vi "RampVoltagewithDDSv12.vi"() -> ()   [LabVIEW 2016]
uses:
  <vilib>/DAQmx/write.llb/DAQmx Write (Digital 1D Wfm NChan NSamp).vi
  <vilib>/DAQmx/write.llb/DAQmx Write (Analog 2D DBL NChan NSamp).vi
  <vilib>/DAQmx/create/channels.llb/DAQmx Create Channel (AO-Voltage-Basic).vi
  <vilib>/DAQmx/create/channels.llb/DAQmx Create Channel (DO-Digital Output).vi
  <vilib>/DAQmx/configure/timing.llb/DAQmx Timing (Sample Clock).vi
  <vilib>/DAQmx/configure/trigger.llb/DAQmx Start Trigger (Digital Edge).vi
  <vilib>/DAQmx/miscellaneous.llb/DAQmx Fill In Error Info.vi
  <vilib>/Waveform/DWDTOps.llb/DWDT Boolean Array to Digital.vi
  <vilib>/Waveform/DWDTOps.llb/DWDT Uncompress Digital.vi
  <vilib>/Waveform/DTblOps.llb/DTbl Digital to Analog.vi
  <resource>/objmgr/daqmx.rc
panel:
  in  "Phase Lock Switch\n(TTL High - Lock Off)":bool
  in  "Phase Lock Switch (Port 0 Line 1)":tag="Dev2/port0/line1"
  out "Digital Output":cluster{i32, dbl, dbl[][]}(graph)={0, 1e-05, [[0.0, 0.0, 0.0, 0.0, 0.0, 0.0, 0.0, 0.0, 0.0, 0.0, 0.0, 0.0, 0.0, 0.0, 0.0, 0.0, 0.0, 0.0, 0.0, 0.0, 0.0, 0.0, 0.0, 0.0, 0.0, 0.0, 0.0, 0.0, 0.0, 0.0, 0.0, 0.0, 0.0, 0.0, 0.0, 0.0, 0.0, 0.0, 0.0, 0.0, 0.0, 0.0, 0.0, 0.0, 0.0, 0.0, 0.0, 0.0, 0.0, 0.0, 0.0, 0.0, 0.0, 0.0, 0.0, 0.0, 0.0, 0.0, 0.0, 0.0, 0.0, 0.0, 0.0, 0.0, 0.0, 0.0, 0.0, 0.0, 0.0, 0.0, 0.0, 0.0, 0.0, 0.0, 0.0, 0.0, 0.0, 0.0, 0.0, 0.0, 0.0, 0.0, 0.0, 0.0, 0.0, 0.0, 0.0, 0.0, 0.0, 0.0, 0.0, 0.0, 0.0, 0.0, 0.0, 0.0, 0.0, 0.0, 0.0, 0.0, 5.0, 5.0, 5.0, 5.0, 5.0, 5.0, 5.0, 5.0, 5.0, 5.0, 5.0, 5.0, 5.0, 5.0, 5.0, 5.0, 5.0, 5.0, 5.0, 5.0, 5.0, 5.0, 5.0, 5.0, 5.0, 5.0, 5.0, 5.0, 5.0, 5.0, 5.0, 5.0, 5.0, 5.0, 5.0, 5.0, 5.0, 5.0, 5.0, 5.0, 5.0, 5.0, 5.0, 5.0, 5.0, 5.0, 5.0, 5.0, 5.0, 5.0, 5.0, 5.0, 5.0, 5.0, 5.0, 5.0, 5.0, 5.0, 5.0, 5.0, 5.0, 5.0, 5.0, 5.0, 5.0, 5.0, 5.0, 5.0, 5.0, 5.0, 5.0, 5.0, 5.0, 5.0, 5.0, 5.0, 5.0, 5.0, 5.0, 5.0, 5.0, 5.0, 5.0, 5.0, 5.0, 5.0, 5.0, 5.0, 5.0, 5.0, 5.0, 5.0, 5.0, 5.0, 5.0, 5.0, 5.0, 5.0, 5.0, 5.0, 5.0, 5.0, 5.0, 5.0, 5.0, 5.0, 5.0, 5.0, 5.0, 5.0, 5.0, 5.0, 5.0, 5.0, 5.0, 5.0, 5.0, 5.0, 5.0, 5.0, 5.0, 5.0, 5.0, 5.0, 5.0, 5.0, 5.0, 5.0, 5.0, 5.0, 5.0, 5.0, 5.0, 5.0, 5.0, 5.0, 5.0, 5.0, 5.0, 5.0, 5.0, 5.0, 5.0, 5.0, 5.0, 5.0, 5.0, 5.0, 5.0, 5.0, 5.0, 5.0, 5.0, 5.0, 5.0, 5.0, 5.0, 5.0, 5.0, 5.0, 5.0, 5.0, 5.0, 5.0, 5.0, 5.0, 5.0, 5.0, 5.0, 5.0, 5.0, 5.0, 5.0, 5.0, 5.0, 5.0, 5.0, 5.0, 5.0, 5.0, 5.0, 5.0, 5.0, 5.0, 5.0, 5.0, 5.0, 5.0, 5.0, 5.0, 5.0, 5.0, 5.0, 5.0, 5.0, 5.0, 5.0, 5.0, 5.0, 5.0, 0.0, 0.0, 0.0, 0.0, 0.0, 0.0, 0.0, 0.0, 0.0, 0.0, 0.0, 0.0, 0.0, 0.0, 0.0, 0.0, 0.0, 0.0, 0.0, 0.0, 0.0, 0.0, 0.0, 0.0, 0.0, 0.0, 0.0, 0.0, 0.0, 0.0, 0.0, 0.0, 0.0, 0.0, 0.0, 0.0, 0.0, 0.0, 0.0, 0.0, 0.0, 0.0, 0.0, 0.0, 0.0, 0.0, 0.0, 0.0, 0.0, 0.0, 0.0, 0.0, 0.0, 0.0, 0.0, 0.0, 0.0, 0.0, 0.0, 0.0, 0.0, 0.0, 0.0, 0.0, 0.0, 0.0, 0.0, 0.0, 0.0, 0.0, 0.0, 0.0, 0.0, 0.0, 0.0, 0.0, 0.0, 0.0, 0.0, 0.0, 0.0, 0.0, 0.0, 0.0, 0.0, 0.0, 0.0, 0.0, 0.0, 0.0, 0.0, 0.0, 0.0, 0.0, 0.0, 0.0, 0.0, 0.0, 0.0, 0.0, 0.0, 0.0, 0.0, 0.0, 0.0, 0.0, 0.0, 0.0, 0.0, 0.0, 0.0, 0.0, 0.0, 0.0, 0.0, 0.0, 0.0, 0.0, 0.0, 0.0, 0.0, 0.0, 0.0, 0.0, 0.0, 0.0, 0.0, 0.0, 0.0, 0.0, 0.0, 0.0, 0.0, 0.0, 0.0, 0.0, 0.0, 0.0, 0.0, 0.0, 0.0, 0.0, 0.0, 0.0, 0.0, 0.0, 0.0, 0.0, 0.0, 0.0, 0.0, 0.0, 0.0, 0.0, 0.0, 0.0, 0.0, 0.0, 0.0, 0.0, 0.0, 0.0, 0.0, 0.0, 0.0, 0.0, 0.0, 0.0, 0.0, 0.0, 0.0, 0.0, 0.0, 0.0, 0.0, 0.0, 0.0, 0.0, 0.0, 0.0, 0.0, 0.0, 0.0, 0.0, 0.0, 0.0, 0.0, 0.0, 0.0, 0.0, 0.0, 0.0, 0.0, 0.0, 0.0, 0.0, 0.0, 0.0, 0.0, 0.0, 5.0, 5.0, 5.0, 5.0, 5.0, 5.0, 5.0, 5.0, 5.0, 5.0, 5.0, 5.0, 5.0, 5.0, 5.0, 5.0, 5.0, 5.0, 5.0, 5.0, 5.0, 5.0, 5.0, 5.0, 5.0, 5.0, 5.0, 5.0, 5.0, 5.0, 5.0, 5.0, 5.0, 5.0, 5.0, 5.0, 5.0, 5.0, 5.0, 5.0, 5.0, 5.0, 5.0, 5.0, 5.0, 5.0, 5.0, 5.0, 5.0, 5.0, 5.0, 5.0, 5.0, 5.0, 5.0, 5.0, 5.0, 5.0, 5.0, 5.0, 5.0, 5.0, 5.0, 5.0, 5.0, 5.0, 5.0, 5.0, 5.0, 5.0, 5.0, 5.0, 5.0, 5.0, 5.0, 5.0, 5.0, 5.0, 5.0, 5.0, 5.0, 5.0, 5.0, 5.0, 5.0, 5.0, 5.0, 5.0, 5.0, 5.0, 5.0, 5.0, 5.0, 5.0, 5.0, 5.0, 5.0, 5.0, 5.0, 5.0, 5.0, 5.0, 5.0, 5.0, 5.0, 5.0, 5.0, 5.0, 5.0, 5.0, 5.0, 5.0, 5.0, 5.0, 5.0, 5.0, 5.0, 5.0, 5.0, 5.0, 5.0, 5.0, 5.0, 5.0, 5.0, 5.0, 5.0, 5.0, 5.0, 5.0, 5.0, 5.0, 5.0, 5.0, 5.0, 5.0, 5.0, 5.0, 5.0, 5.0, 5.0, 5.0, 5.0, 5.0, 5.0, 5.0, 5.0, 5.0, 5.0, 5.0, 5.0, 5.0, 5.0, 5.0, 5.0, 5.0, 5.0, 5.0, 5.0, 5.0, 5.0, 5.0, 5.0, 5.0, 5.0, 5.0, 5.0, 5.0, 5.0, 5.0, 5.0, 5.0, 5.0, 5.0, 5.0, 5.0, 5.0, 5.0, 5.0, 5.0, 5.0, 5.0, 5.0, 5.0, 5.0, 5.0, 5.0, 5.0, 5.0, 5.0, 5.0, 5.0, 5.0, 5.0, 5.0, 5.0, 5.0, 5.0, 5.0, 5.0, 0.0, 0.0, 0.0, 0.0, 0.0, 0.0, 0.0, 0.0, 0.0, 0.0, 0.0, 0.0, 0.0, 0.0, 0.0, 0.0, 0.0, 0.0, 0.0, 0.0, 0.0, 0.0, 0.0, 0.0, 0.0, 0.0, 0.0, 0.0, 0.0, 0.0, 0.0, 0.0, 0.0, 0.0, 0.0, 0.0, 0.0, 0.0, 0.0, 0.0, 0.0, 0.0, 0.0, 0.0, 0.0, 0.0, 0.0, 0.0, 0.0, 0.0, 0.0, 0.0, 0.0, 0.0, 0.0, 0.0, 0.0, 0.0, 0.0, 0.0, 0.0, 0.0, 0.0, 0.0, 0.0, 0.0, 0.0, 0.0, 0.0, 0.0, 0.0, 0.0, 0.0, 0.0, 0.0, 0.0, 0.0, 0.0, 0.0, 0.0, 0.0, 0.0, 0.0, 0.0, 0.0, 0.0, 0.0, 0.0, 0.0, 0.0, 0.0, 0.0, 0.0, 0.0, 0.0, 0.0, 0.0, 0.0, 0.0, 0.0, 5.0], [5.0, 5.0, 5.0, 5.0, 5.0, 5.0, 5.0, 5.0, 5.0, 5.0, 5.0, 5.0, 5.0, 5.0, 5.0, 5.0, 5.0, 5.0, 5.0, 5.0, 5.0, 5.0, 5.0, 5.0, 5.0, 5.0, 5.0, 5.0, 5.0, 5.0, 5.0, 5.0, 5.0, 5.0, 5.0, 5.0, 5.0, 5.0, 5.0, 5.0, 5.0, 5.0, 5.0, 5.0, 5.0, 5.0, 5.0, 5.0, 5.0, 5.0, 5.0, 5.0, 5.0, 5.0, 5.0, 5.0, 5.0, 5.0, 5.0, 5.0, 5.0, 5.0, 5.0, 5.0, 5.0, 5.0, 5.0, 5.0, 5.0, 5.0, 5.0, 5.0, 5.0, 5.0, 5.0, 5.0, 5.0, 5.0, 5.0, 5.0, 5.0, 5.0, 5.0, 5.0, 5.0, 5.0, 5.0, 5.0, 5.0, 5.0, 5.0, 5.0, 5.0, 5.0, 5.0, 5.0, 5.0, 5.0, 5.0, 5.0, 5.0, 5.0, 5.0, 5.0, 5.0, 5.0, 5.0, 5.0, 5.0, 5.0, 5.0, 5.0, 5.0, 5.0, 5.0, 5.0, 5.0, 5.0, 5.0, 5.0, 5.0, 5.0, 5.0, 5.0, 5.0, 5.0, 5.0, 5.0, 5.0, 5.0, 5.0, 5.0, 5.0, 5.0, 5.0, 5.0, 5.0, 5.0, 5.0, 5.0, 5.0, 5.0, 5.0, 5.0, 5.0, 5.0, 5.0, 5.0, 5.0, 5.0, 0.0, 0.0, 0.0, 0.0, 0.0, 0.0, 0.0, 0.0, 0.0, 0.0, 0.0, 0.0, 0.0, 0.0, 0.0, 0.0, 0.0, 0.0, 0.0, 0.0, 0.0, 0.0, 0.0, 0.0, 0.0, 0.0, 0.0, 0.0, 0.0, 0.0, 0.0, 0.0, 0.0, 0.0, 0.0, 0.0, 0.0, 0.0, 0.0, 0.0, 0.0, 0.0, 0.0, 0.0, 0.0, 0.0, 0.0, 0.0, 0.0, 0.0, 0.0, 0.0, 0.0, 0.0, 0.0, 0.0, 0.0, 0.0, 0.0, 0.0, 0.0, 0.0, 0.0, 0.0, 0.0, 0.0, 0.0, 0.0, 0.0, 0.0, 0.0, 0.0, 0.0, 0.0, 0.0, 0.0, 0.0, 0.0, 0.0, 0.0, 0.0, 0.0, 0.0, 0.0, 0.0, 0.0, 0.0, 0.0, 0.0, 0.0, 0.0, 0.0, 0.0, 0.0, 0.0, 0.0, 0.0, 0.0, 0.0, 0.0, 0.0, 0.0, 0.0, 0.0, 0.0, 0.0, 0.0, 0.0, 0.0, 0.0, 0.0, 0.0, 0.0, 0.0, 0.0, 0.0, 0.0, 0.0, 0.0, 0.0, 0.0, 0.0, 0.0, 0.0, 0.0, 0.0, 0.0, 0.0, 0.0, 0.0, 0.0, 0.0, 0.0, 0.0, 0.0, 0.0, 0.0, 0.0, 0.0, 0.0, 0.0, 0.0, 0.0, 0.0, 0.0, 0.0, 0.0, 0.0, 0.0, 0.0, 0.0, 0.0, 0.0, 0.0, 0.0, 0.0, 0.0, 0.0, 0.0, 0.0, 0.0, 0.0, 0.0, 0.0, 0.0, 0.0, 0.0, 0.0, 0.0, 0.0, 0.0, 0.0, 0.0, 0.0, 0.0, 0.0, 0.0, 0.0, 0.0, 0.0, 0.0, 0.0, 0.0, 0.0, 0.0, 0.0, 0.0, 0.0, 0.0, 0.0, 0.0, 0.0, 0.0, 0.0, 0.0, 0.0, 0.0, 0.0, 0.0, 0.0, 0.0, 0.0, 0.0, 0.0, 0.0, 0.0, 0.0, 0.0, 0.0, 0.0, 0.0, 0.0, 0.0, 0.0, 0.0, 0.0, 0.0, 0.0, 0.0, 0.0, 0.0, 0.0, 0.0, 0.0, 0.0, 0.0, 0.0, 0.0, 0.0, 0.0, 0.0, 0.0, 0.0, 0.0, 0.0, 0.0, 0.0, 0.0, 0.0, 0.0, 0.0, 0.0, 0.0, 0.0, 0.0, 0.0, 0.0, 0.0, 0.0, 0.0, 0.0, 0.0, 0.0, 0.0, 0.0, 0.0, 0.0, 0.0, 0.0, 0.0, 0.0, 0.0, 0.0, 0.0, 0.0, 0.0, 0.0, 0.0, 0.0, 0.0, 0.0, 0.0, 0.0, 0.0, 0.0, 0.0, 0.0, 0.0, 0.0, 0.0, 0.0, 0.0, 0.0, 0.0, 0.0, 0.0, 0.0, 0.0, 0.0, 0.0, 0.0, 0.0, 0.0, 0.0, 0.0, 0.0, 0.0, 0.0, 0.0, 0.0, 0.0, 0.0, 0.0, 0.0, 0.0, 0.0, 0.0, 0.0, 0.0, 0.0, 0.0, 0.0, 0.0, 0.0, 0.0, 0.0, 0.0, 0.0, 0.0, 0.0, 0.0, 0.0, 0.0, 0.0, 0.0, 0.0, 0.0, 0.0, 0.0, 0.0, 0.0, 0.0, 0.0, 0.0, 0.0, 0.0, 0.0, 0.0, 0.0, 0.0, 0.0, 0.0, 0.0, 0.0, 0.0, 0.0, 0.0, 0.0, 0.0, 0.0, 0.0, 0.0, 0.0, 0.0, 0.0, 0.0, 0.0, 0.0, 0.0, 0.0, 0.0, 0.0, 0.0, 0.0, 0.0, 0.0, 0.0, 0.0, 0.0, 0.0, 0.0, 0.0, 0.0, 0.0, 0.0, 0.0, 0.0, 0.0, 0.0, 0.0, 0.0, 0.0, 0.0, 0.0, 0.0, 0.0, 0.0, 0.0, 0.0, 0.0, 0.0, 0.0, 0.0, 0.0, 0.0, 0.0, 0.0, 0.0, 0.0, 0.0, 0.0, 0.0, 0.0, 0.0, 0.0, 0.0, 0.0, 0.0, 0.0, 0.0, 0.0, 0.0, 0.0, 0.0, 0.0, 0.0, 0.0, 0.0, 0.0, 0.0, 0.0, 0.0, 0.0, 0.0, 0.0, 0.0, 0.0, 0.0, 0.0, 0.0, 0.0, 0.0, 0.0, 0.0, 0.0, 0.0, 0.0, 0.0, 0.0, 0.0, 0.0, 0.0, 0.0, 0.0, 0.0, 0.0, 0.0, 0.0, 0.0, 0.0, 0.0, 0.0, 0.0, 0.0, 0.0, 0.0, 0.0, 0.0, 0.0, 0.0, 0.0, 0.0, 0.0, 0.0, 0.0, 0.0, 0.0, 0.0, 0.0, 0.0, 0.0, 0.0, 0.0, 0.0, 0.0, 0.0, 0.0, 0.0, 0.0, 0.0, 0.0, 0.0, 0.0, 0.0, 0.0, 0.0, 0.0, 0.0, 0.0, 0.0, 0.0, 0.0, 0.0, 0.0, 0.0, 0.0, 0.0, 0.0, 0.0, 0.0, 0.0, 0.0, 0.0, 0.0, 0.0, 0.0, 0.0, 0.0, 0.0, 0.0, 0.0, 0.0, 0.0, 0.0, 0.0, 0.0, 0.0, 0.0, 0.0, 0.0, 0.0, 0.0, 0.0, 0.0, 0.0, 0.0, 0.0, 0.0, 0.0, 0.0, 0.0, 0.0, 0.0, 0.0, 0.0, 0.0, 0.0, 0.0, 0.0, 0.0, 0.0, 0.0, 0.0, 0.0, 0.0, 0.0, 0.0, 0.0, 0.0, 0.0, 0.0, 0.0, 0.0, 0.0, 0.0, 0.0, 0.0, 0.0, 0.0, 0.0, 0.0, 0.0, 0.0, 0.0, 0.0, 0.0, 0.0, 0.0, 0.0, 0.0, 0.0, 0.0, 0.0, 0.0, 0.0, 0.0, 0.0, 0.0, 0.0, 0.0, 0.0, 0.0, 0.0, 0.0, 0.0, 0.0, 0.0, 0.0, 0.0, 0.0, 0.0, 0.0, 0.0, 0.0, 0.0, 0.0, 0.0, 0.0, 0.0, 0.0, 0.0, 0.0, 0.0, 0.0, 0.0, 0.0, 0.0, 0.0, 0.0, 0.0, 0.0, 0.0, 0.0, 0.0, 0.0, 0.0, 0.0, 0.0, 0.0, 0.0, 0.0, 0.0, 0.0, 0.0, 0.0, 0.0, 0.0, 0.0, 0.0, 0.0, 0.0, 0.0, 0.0, 0.0, 0.0, 0.0, 0.0, 0.0, 0.0, 0.0, 0.0, 0.0, 0.0, 0.0, 0.0, 0.0, 0.0, 0.0, 0.0, 0.0, 5.0]]}
  out "Analog Outputs":cluster{i32, dbl, dbl[][]}(graph)={0, 4e-06, array4x2001[8004 elements]}
  in  "DDS Trigger (Port 0 Line 0)":tag="Dev2/port0/line0"
  in  "DDS trigger delay (ms)":dbl step=0.01
  in  "error in 2":errorcluster caption="error in"
  in  "ao3 ramp amplitude (V)":dbl
  in  "ao2 ramp amplitude (V)":dbl
  in  "ao1 ramp amplitude (V)":dbl
  in  "SolsTiS 2 - Fast Piezo (ao3)":tag="Dev2/ao3"
  in  "SolsTiS 2 - Slow Piezo (ao2)":tag="Dev2/ao2"
  out "size(s)":i32=2001
  in  "Trigger delay NI (ms)":dbl=1.0
  in  "Trigger Input (PFI0)":tag="/Dev2/PFI0"
  in  "SolsTiS 1 - Fast Piezo (ao1)":tag="Dev2/ao1"
  in  "SolsTiS 1 - Slow Piezo (ao0)":tag="Dev2/ao0"
  in  "Plateau duration (ms)":dbl=2.0 step=0.01
  in  "Ramp duration (ms)":dbl=2.0 step=0.01
  in  "ao0 ramp amplitude (V)":dbl=0.09 step=0.001
  in  "error in":errorcluster
  # "MAGIS LASER SYSTEM\nChirp Control"
  # "Ramp Definition"
  # "Output Monitor"
  # "Channel Definition"
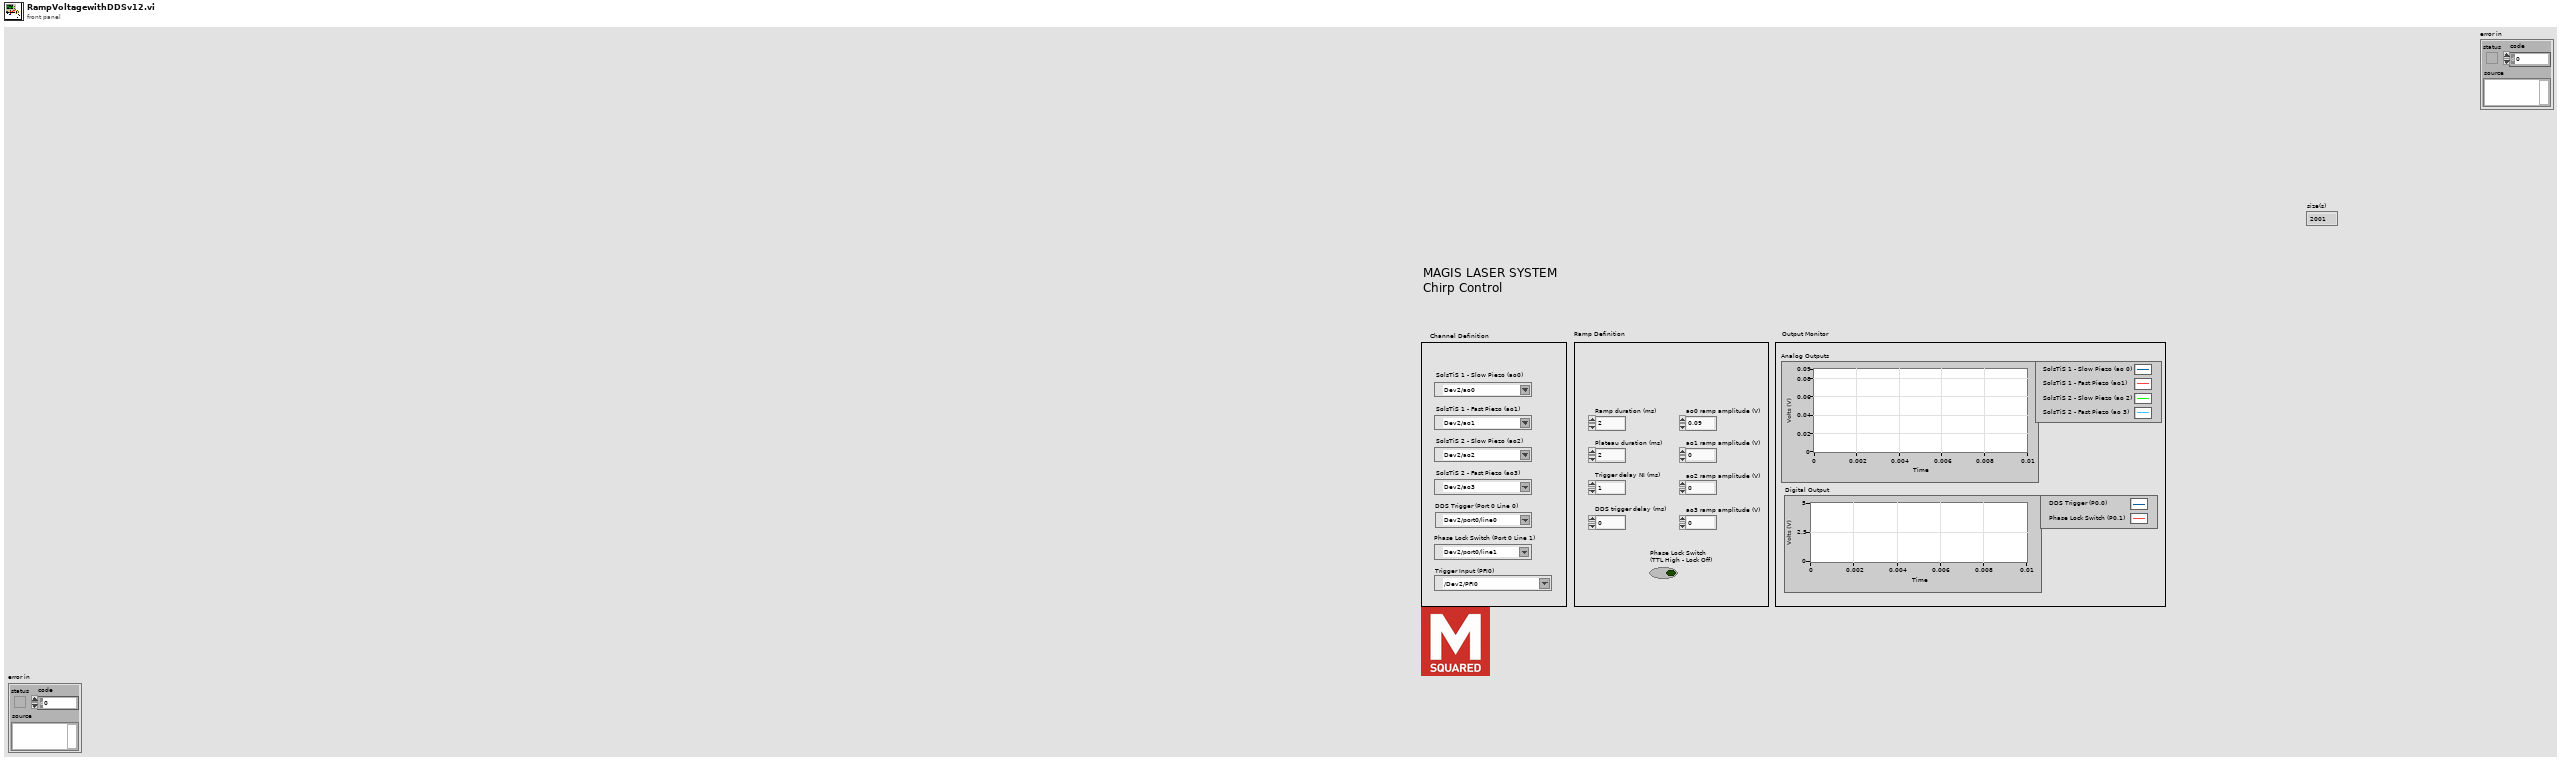
[diagram p1: front panel]
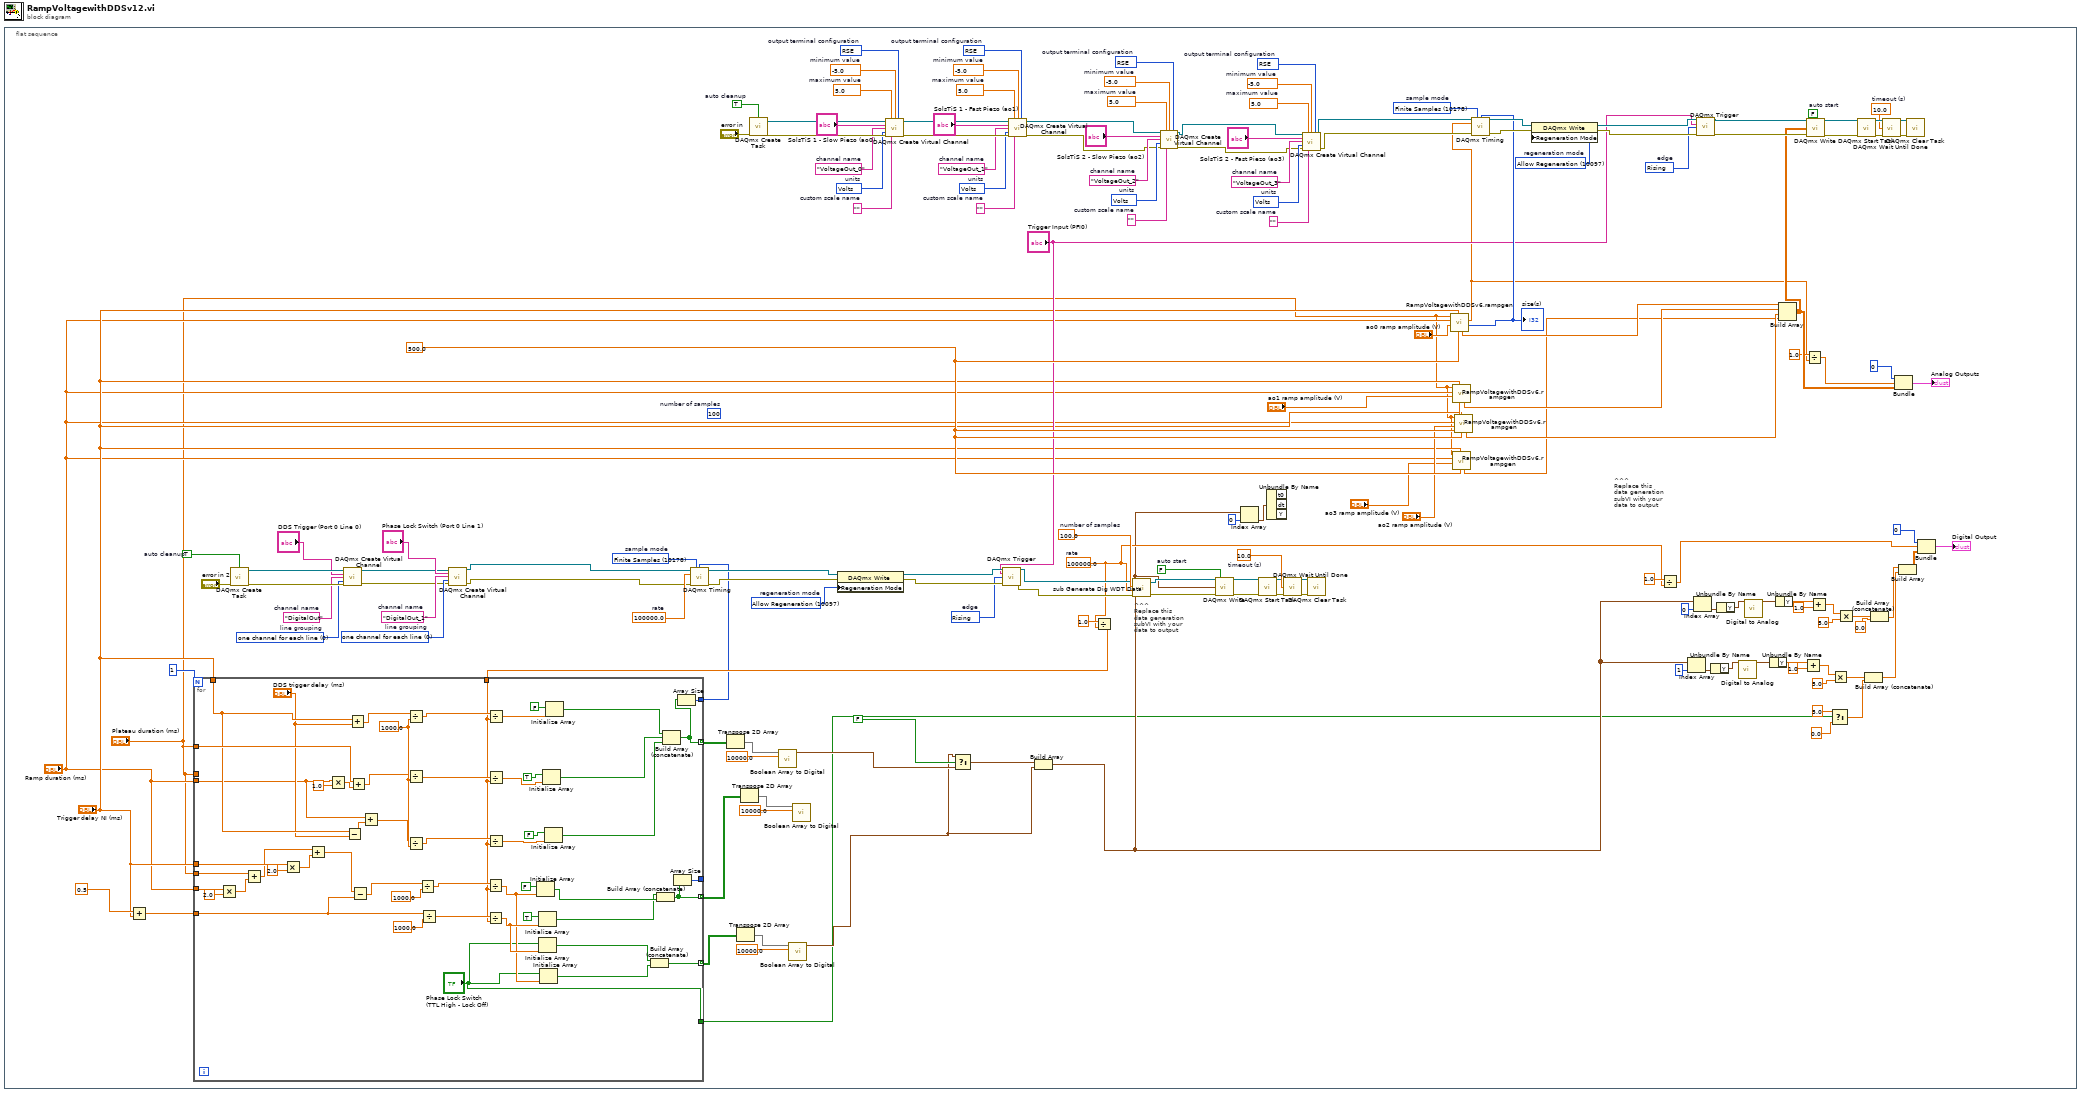
[diagram p0: block diagram]
diagram:
  n1 = flat-sequence {
    frame #0 {
      w38 = 0 items=["one channel for each line", "one channel for all lines"]  # line grouping
      w37 = "DigitalOut_1"  # channel name
      w105 = 500.0 ("No of samples in ramp (500 or less)")
      w72 = 10280 items=["Rising"=10280, "Falling"=10171]  # edge
      w74 = 10097 items=["Allow Regeneration"=10097, "Do Not Allow Regeneration"=10158]  # regeneration mode
      w77 = 10178 items=["Finite Samples"=10178, "Continuous Samples"=10123, "Hardware Timed Single Point"=12522]  # sample mode
      (unwired) 100  # number of samples
      w78 = 100000.0  # rate
      w81 = 0 items=["one channel for each line", "one channel for all lines"]  # line grouping
      w80 = "DigitalOut"  # channel name
      w83 = TRUE  # auto cleanup
      w98 = 10.0  # timeout (s)
      w46 = 100000.0  # rate
      w91 = 100.0  # number of samples
      w88 = FALSE  # auto start
      w112 = 10083 items=["Default"=-1, "RSE"=10083, "Differential"=10106, "Pseudodifferential"=12529]  # output terminal configuration
      w113 = 10348 items=["Volts"=10348, "From Custom Scale"=10065]  # units
      w114 = "VoltageOut_3"  # channel name
      w115 = ""  # custom scale name
      w116 = -5.0  # minimum value
      w117 = 5.0  # maximum value
      w121 = 10083 items=["Default"=-1, "RSE"=10083, "Differential"=10106, "Pseudodifferential"=12529]  # output terminal configuration
      w122 = 10348 items=["Volts"=10348, "From Custom Scale"=10065]  # units
      w123 = "VoltageOut_2"  # channel name
      w124 = ""  # custom scale name
      w125 = -5.0  # minimum value
      w126 = 5.0  # maximum value
      w133 = 10280 items=["Rising"=10280, "Falling"=10171]  # edge
      w135 = 10097 items=["Allow Regeneration"=10097, "Do Not Allow Regeneration"=10158]  # regeneration mode
      w138 = 10178 items=["Finite Samples"=10178, "Continuous Samples"=10123, "Hardware Timed Single Point"=12522]  # sample mode
      w140 = 10083 items=["Default"=-1, "RSE"=10083, "Differential"=10106, "Pseudodifferential"=12529]  # output terminal configuration
      w141 = 10348 items=["Volts"=10348, "From Custom Scale"=10065]  # units
      w142 = "VoltageOut_1"  # channel name
      w143 = ""  # custom scale name
      w144 = -5.0  # minimum value
      w145 = 5.0  # maximum value
      w147 = 10083 items=["Default"=-1, "RSE"=10083, "Differential"=10106, "Pseudodifferential"=12529]  # output terminal configuration
      w148 = 10348 items=["Volts"=10348, "From Custom Scale"=10065]  # units
      w149 = "VoltageOut_0"  # channel name
      w151 = ""  # custom scale name
      w152 = -5.0  # minimum value
      w153 = 5.0  # maximum value
      w155 = TRUE  # auto cleanup
      w161 = 10.0  # timeout (s)
      w165 = FALSE  # auto start
      # "^^^\nReplace this\ndata generation\nsubVI with your\ndata to output"
      # "^^^\nReplace this\ndata generation\nsubVI with your\ndata to output"
      n2 = Add(x=0.5 ("DDS Trigger delay (ms)"), y="Trigger delay NI (ms)") -> (x+y=w32:dbl)
      n3 = call <vilib>:"DAQmx Create Task.vi"("auto cleanup"=w83, "error in"="error in 2") -> ("task out"=w82:refnum<k21>, "error out"=w84:errorcluster)  [unwired: 12 in]
      n4 = call-poly <vilib>:"DAQmx Create Virtual Channel.vi"("task in"=w82, "lines"="DDS Trigger (Port 0 Line 0)", "name to assign"=w80, "line grouping"=w81, "error in"=w84) -> ("task out"=w34:refnum<k21>, "error out"=w35:errorcluster)  [unwired: 9 in]
      n5 = call-poly <vilib>:"DAQmx Create Virtual Channel.vi"("task in"=w34, "lines"="Phase Lock Switch (Port 0 Line 1)", "name to assign"=w37, "line grouping"=w38, "error in"=w35) -> ("task out"=w10:refnum<k21>, "error out"=w9:errorcluster)  [unwired: 9 in]
      n6 = call <vilib>:"DAQmx Create Task.vi"("auto cleanup"=w155, "error in"="error in") -> ("task out"=w154:refnum<k21>, "error out"=w156:errorcluster)  [unwired: 12 in]
      n7 = call-poly <vilib>:"DAQmx Create Virtual Channel.vi"("task in"=w154, "maximum value"=w153, "minimum value"=w152, "output terminal configuration"=w147, "physical channels"="SolsTiS 1 - Slow Piezo (ao0)", "name to assign"=w149, "units"=w148, "error in"=w156, "custom scale name"=w151) -> ("task out"=w146:refnum<k21>, "error out"=w150:errorcluster)  [unwired: 5 in]
      n8 = call-poly <vilib>:"DAQmx Create Virtual Channel.vi"("task in"=w146, "maximum value"=w145, "minimum value"=w144, "output terminal configuration"=w140, "physical channels"="SolsTiS 1 - Fast Piezo (ao1)", "name to assign"=w142, "units"=w141, "error in"=w150, "custom scale name"=w143) -> ("task out"=w119:refnum<k21>, "error out"=w118:errorcluster)  [unwired: 5 in]
      n9 = Divide(x=1.0, y=w46) -> (x/y=w68:dbl)
      n10 = for {
        N: 1 -> [_]
        tunnel: w68 -> [w192]
        tunnel: [w207] -> w65 mode=indexing
        tunnel: [w206] -> w64
        tunnel: "Plateau duration (ms)" -> [_]
        tunnel: "Trigger delay NI (ms)" -> [w171]
        tunnel: w32 -> [w198]
        tunnel: "Ramp duration (ms)" -> [w202]
        tunnel: "Plateau duration (ms)" -> [w199]
        tunnel: [w189] -> _
        tunnel: "Trigger delay NI (ms)" -> [w186]
        tunnel: [w183] -> w28 mode=indexing
        tunnel: [w179] -> w25 mode=indexing
        tunnel: "Ramp duration (ms)" -> [w168]
        tunnel: "Plateau duration (ms)" -> [w173]
        tunnel: ["Phase Lock Switch\n(TTL High - Lock Off)"] -> w5
        w217 = 1000.0
        n11 = Multiply(x=w202, y=2.0) -> (x*y=w200:dbl)
        n12 = Add(x=w199, y=w200) -> (x+y=w185:dbl)
        n13 = Multiply(x=w186, y=2.0) -> (x*y=w187:dbl)
        n14 = Add(x=w185, y=w187) -> (x+y=w184:dbl)
        n15 = Multiply(x=w168, y=1.0) -> (x*y=w174:dbl)
        n16 = Subtract(x=w171, y="DDS trigger delay (ms)") -> (x-y=w167:dbl)
        n17 = Add(x=w171, y="DDS trigger delay (ms)") -> (x+y=w205:dbl)
        n18 = Add(x=w173, y=w174) -> (x+y=w172:dbl)
        n19 = Subtract(x=w184, y=w198) -> (x-y=w195:dbl)
        n20 = Add(x=w168, y=w167) -> (x+y=w166:dbl)
        n21 = Divide(x=w205, y=w217) -> (x/y=w216:dbl)
        n22 = Divide(x=w172, y=w217) -> (x/y=w215:dbl)
        n23 = Divide(x=w166, y=w217) -> (x/y=w214:dbl)
        n24 = Divide(x=w195, y=1000.0) -> (x/y=w194:dbl)
        n25 = Divide(x=w198, y=1000.0) -> (x/y=w193:dbl)
        n26 = Divide(x=w194, y=w192) -> (x/y=w178:dbl)
        n27 = Divide(x=w193, y=w192) -> (x/y=w182:dbl)
        n28 = Divide(x=w216, y=w192) -> (x/y=w211:dbl)
        n29 = Divide(x=w215, y=w192) -> (x/y=w210:dbl)
        n30 = Divide(x=w214, y=w192) -> (x/y=w209:dbl)
        n31 = Initialize Array(FALSE, w178) -> (w191:bool[])
        n32 = Initialize Array(TRUE, w182) -> (w190:bool[])
        n33 = Initialize Array("Phase Lock Switch\n(TTL High - Lock Off)", w182) -> (w181:bool[])
        n34 = Initialize Array("Phase Lock Switch\n(TTL High - Lock Off)", w178) -> (w180:bool[])
        n35 = Initialize Array(TRUE, w210) -> (w177:bool[])
        n36 = Initialize Array(FALSE, w209) -> (w176:bool[])
        n37 = Initialize Array(FALSE, w211) -> (w208:bool[])
        n38 = Build Array (concatenate)(w181, w180) -> (w179:bool[])
        n39 = Build Array (concatenate)(w190, w191) -> (w183:bool[])
        n40 = Build Array (concatenate)(w208, w177, w176) -> (w207:bool[])
        n41 = Array Size(array=w183) -> (size(s)=w189:i32)
        n42 = Array Size(array=w207) -> (size(s)=w206:i32)
      }
      n43 = call-poly <vilib>:"DAQmx Timing.vi"("task/channels in"=w10, "sample mode"=w77, "samples per channel"=w64, "rate"=w78, "error in"=w9) -> ("task out"=w76:refnum<k21>, "error out"=w79:errorcluster)  [unwired: 9 in]
      n44 = Transpose 2D Array(2D array=w65) -> (transposed array=w66:bool[][])
      n45 = Transpose 2D Array(2D array=w25) -> (transposed array=w26:bool[][])
      n46 = Transpose 2D Array(2D array=w28) -> (transposed array=w29:bool[][])
      n47 = call-poly <vilib>:"Boolean Array to Digital.vi"("sample rate"=10000.0, "boolean array"=w66) -> ("digital waveform"=w14:digitalwaveform)  [unwired: 8 in, 1 out]
      n48 = call-poly <vilib>:"Boolean Array to Digital.vi"("sample rate"=10000.0, "boolean array"=w26) -> ("digital waveform"=w6:digitalwaveform)  [unwired: 8 in, 1 out]
      n49 = call-poly <vilib>:"Boolean Array to Digital.vi"("sample rate"=10000.0, "boolean array"=w29) -> ()  [unwired: 8 in, 2 out]
      n50 = property class="DAQmx Write"(reference=w76, error in=w79, "Regeneration Mode"=w74) -> (reference out=w73:refnum<k21>, error out=w75:errorcluster)
      n51 = Select(t=w6, s=FALSE ("Constant PO.0?"), f=w14) -> (s? t:f=w12:digitalwaveform)
      n52 = call-poly <vilib>:"DAQmx Trigger.vi"("task/channels in"=w73, "source"="Trigger Input (PFI0)", "edge"=w72, "error in"=w75) -> ("task out"=w71:refnum<k21>, "error out"=w70:errorcluster)  [unwired: 10 in]
      n53 = Build Array(w12, w6) -> (w11:digitalwaveform[])
      n54 = call <vilib>:"sub Generate Dig WDT Data.vi"("task in"=w71, "number of samples"=w91, "update rate"=w46, "error in"=w70) -> ("task out"=w90:refnum<k21>, "error out"=w89:errorcluster)  [unwired: 1 in, 1 out]
      n55 = call-poly <vilib>:"DAQmx Create Virtual Channel.vi"("task in"=w119, "maximum value"=w126, "minimum value"=w125, "output terminal configuration"=w121, "physical channels"="SolsTiS 2 - Slow Piezo (ao2)", "name to assign"=w123, "units"=w122, "error in"=w118, "custom scale name"=w124) -> ("task out"=w110:refnum<k21>, "error out"=w109:errorcluster)  [unwired: 5 in]
      n56 = call-poly <vilib>:"DAQmx Write.vi"("task/channels in"=w90, "auto start"=w88, "data"=w11, "error in"=w89) -> ("task out"=w95:refnum<k21>, "error out"=w96:errorcluster)  [unwired: 9 in, 1 out]
      n57 = Index Array(array=w11, index=0) -> (element=w86:digitalwaveform)
      n58 = call <vilib>:"DAQmx Start Task.vi"("task/channels in"=w95, "error in"=w96) -> ("task out"=w92:refnum<k21>, "error out"=w93:errorcluster)  [unwired: 12 in]
      n59 = Unbundle By Name(w86) -> ()  [unwired: 3 out]
      n60 = call <vilib>:"DAQmx Wait Until Done.vi"("task/channels in"=w92, "timeout (sec)"=w98, "error in"=w93) -> ("task out"=w97:refnum<k21>, "error out"=w94:errorcluster)  [unwired: 11 in]
      n61 = call-poly <vilib>:"DAQmx Create Virtual Channel.vi"("task in"=w110, "maximum value"=w117, "minimum value"=w116, "output terminal configuration"=w112, "physical channels"="SolsTiS 2 - Fast Piezo (ao3)", "name to assign"=w114, "units"=w113, "error in"=w109, "custom scale name"=w115) -> ("task out"=w107:refnum<k21>, "error out"=w108:errorcluster)  [unwired: 5 in]
      n62 = call <vilib>:"DAQmx Clear Task.vi"("task in"=w97, "error in"=w94) -> ()  [unwired: 13 in, 1 out]
      n63 = call "RampVoltagewithDDSv6,rampgen.vi"("No of samples in ramp"=w105, "Trigger delay NI (ms)"="Trigger delay NI (ms)", "Ramp Amplitude (V)}"="ao0 ramp amplitude (V)", "Ramp duration (ms)"="Ramp duration (ms)", "Plateau duration (ms)"="Plateau duration (ms)") -> ("Numeric 2"=w129:i32, "Numeric"=w49:dbl, "Array"=w106:dbl[])  [unwired: 3 in, 1 out]
      "size(s)" <- w129
      n64 = call "RampVoltagewithDDSv6,rampgen.vi"("No of samples in ramp"=w105, "Trigger delay NI (ms)"="Trigger delay NI (ms)", "Ramp Amplitude (V)}"="ao1 ramp amplitude (V)", "Ramp duration (ms)"="Ramp duration (ms)", "Plateau duration (ms)"="Plateau duration (ms)") -> ("Array"=w101:dbl[])  [unwired: 3 in, 3 out]
      n65 = call "RampVoltagewithDDSv6,rampgen.vi"("No of samples in ramp"=w105, "Trigger delay NI (ms)"="Trigger delay NI (ms)", "Ramp Amplitude (V)}"="ao3 ramp amplitude (V)", "Ramp duration (ms)"="Ramp duration (ms)", "Plateau duration (ms)"="Plateau duration (ms)") -> ("Array"=w99:dbl[])  [unwired: 3 in, 3 out]
      n66 = call "RampVoltagewithDDSv6,rampgen.vi"("No of samples in ramp"=w105, "Trigger delay NI (ms)"="Trigger delay NI (ms)", "Ramp Amplitude (V)}"="ao2 ramp amplitude (V)", "Ramp duration (ms)"="Ramp duration (ms)", "Plateau duration (ms)"="Plateau duration (ms)") -> ("Array"=w100:dbl[])  [unwired: 3 in, 3 out]
      n67 = call-poly <vilib>:"DAQmx Timing.vi"("task/channels in"=w107, "sample mode"=w138, "samples per channel"=w129, "rate"=w49, "error in"=w108) -> ("task out"=w137:refnum<k21>, "error out"=w139:errorcluster)  [unwired: 9 in]
      n68 = property class="DAQmx Write"(reference=w137, error in=w139, "Regeneration Mode"=w135) -> (reference out=w134:refnum<k21>, error out=w136:errorcluster)
      n69 = Divide(x=1.0, y=w46) -> (x/y=w45:dbl)
      n70 = Index Array(array=w11, index=1) -> (element=w23:digitalwaveform)
      n71 = Index Array(array=w11, index=0) -> (element=w56:digitalwaveform)
      n72 = call-poly <vilib>:"DAQmx Trigger.vi"("task/channels in"=w134, "source"="Trigger Input (PFI0)", "edge"=w133, "error in"=w136) -> ("task out"=w131:refnum<k21>, "error out"=w130:errorcluster)  [unwired: 10 in]
      n73 = Unbundle By Name(w23) -> ("Y"=w22:digitaldata)
      n74 = Unbundle By Name(w56) -> ("Y"=w55:digitaldata)
      n75 = call-poly <vilib>:"Digital to Analog.vi"("digital table"=w22) -> ("analog waveform"=w21:waveform(dbl))  [unwired: 7 in, 3 out]
      n76 = call-poly <vilib>:"Digital to Analog.vi"("digital table"=w55) -> ("analog waveform"=w54:waveform(dbl))  [unwired: 7 in, 3 out]
      n77 = Unbundle By Name(w21) -> ("Y"=w19:dbl[])
      n78 = Unbundle By Name(w54) -> ("Y"=w43:dbl[])
      n79 = Build Array(w106, w101, w100, w99) -> (w60:dbl[][])
      n80 = Add(x=w19, y=1.0) -> (x+y=w18:dbl[])
      n81 = Divide(x=1.0, y=w49) -> (x/y=w48:dbl)
      n82 = call-poly <vilib>:"DAQmx Write.vi"("task/channels in"=w131, "auto start"=w165, "data"=w60, "error in"=w130) -> ("task out"=w160:refnum<k21>, "error out"=w159:errorcluster)  [unwired: 9 in, 1 out]
      n83 = Add(x=w43, y=1.0) -> (x+y=w42:dbl[])
      n84 = Select(t=5.0, s=w5, f=0.0 ("y")) -> (s? t:f=w2:dbl)
      n85 = Multiply(x=w18, y=5.0) -> (x*y=w16:dbl[])
      n86 = Multiply(x=w42, y=5.0) -> (x*y=w40:dbl[])
      n87 = call <vilib>:"DAQmx Start Task.vi"("task/channels in"=w160, "error in"=w159) -> ("task out"=w164:refnum<k21>, "error out"=w163:errorcluster)  [unwired: 12 in]
      n88 = Build Array (concatenate)(w16, w2) -> (w15:dbl[])
      n89 = Build Array (concatenate)(w40, 0.0 ("y")) -> (w39:dbl[])
      n90 = call <vilib>:"DAQmx Wait Until Done.vi"("task/channels in"=w164, "timeout (sec)"=w161, "error in"=w163) -> ("task out"=w158:refnum<k21>, "error out"=w162:errorcluster)  [unwired: 11 in]
      n91 = Bundle(0, w48, w60) -> (→"Analog Outputs":cluster{i32, dbl, dbl[][]})  [unwired: 1 in]
      n92 = Build Array(w39, w15) -> (w51:dbl[][])
      n93 = call <vilib>:"DAQmx Clear Task.vi"("task in"=w158, "error in"=w162) -> ()  [unwired: 13 in, 1 out]
      n94 = Bundle(0, w45, w51) -> (→"Digital Output":cluster{i32, dbl, dbl[][]})  [unwired: 1 in]
    }
  }
